vi "cleanPhaseSpaceData (SubVI).vi"(5 "raw trigger":dbl[][](array[numeric]), 7 "raw time":dbl[](array[numeric]), 8 "raw data":dbl[][](array[numeric])) -> (0 "data":waveform(dbl)[](array[waveform]), 1 "time stamp":dbl[](array[numeric]), 2 "stamped data":dbl[][](array[numeric]), 3 "raw data":dbl[][](array[numeric]), 4 "trigger PS":dbl[][](array[numeric]))   [LabVIEW 2017]
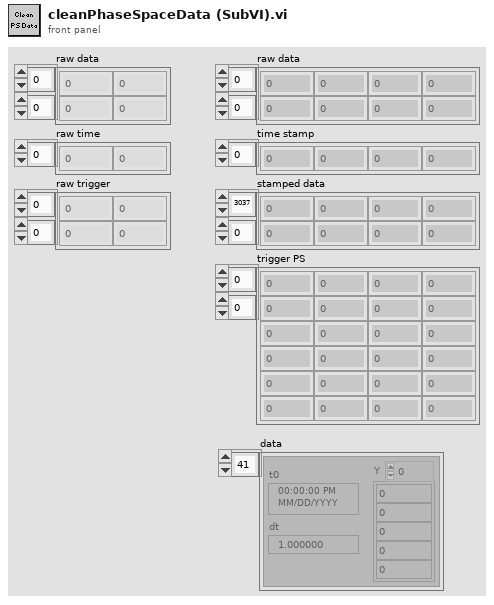
[diagram p1: front panel]
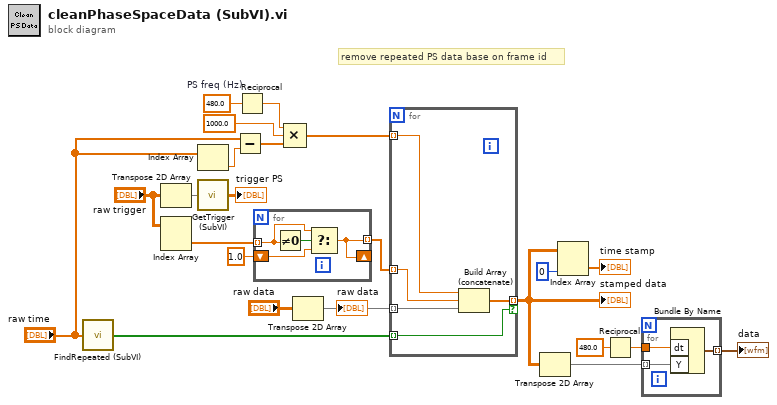
[diagram p0: block diagram]
diagram:
  w19 = 480.0  # PS freq (Hz)
  # "remove repeated PS data base on frame id"
  n1 = call "FindRepeated (SubVI).vi"("time stamp"="raw time") -> ("not repeated?"=w22:bool[])
  n2 = Transpose 2D Array(2D array="raw trigger") -> (transposed array=w14:dbl[][])
  n3 = Index Array(array="raw trigger") -> (element=w3:dbl[])  [unwired: 2 in]
  n4 = Index Array(array="raw time") -> (element=w17:dbl)  [unwired: 1 in]
  n5 = call "GetTrigger (SubVI).vi"("Array in"=w14) -> ("Array out"=→"trigger PS":dbl[][])  [unwired: 4 in]
  n6 = Subtract(x="raw time", y=w17) -> (x-y=w18:dbl[])
  n7 = Reciprocal(x=w19) -> (1/x=w20:dbl)
  n8 = for {
    tunnel: w3 -> [w26] mode=indexing
    shift-right: [w24] -> _
    shift-left: 1.0 -> [w25]
    tunnel: [w24] -> w1 mode=indexing
    n9 = Not Equal To 0?(x=w26) -> (x != 0?=w27:bool)
    n10 = Select(t=w26, s=w27, f=w25) -> (s? t:f=w24:dbl)
  }
  n11 = Compound Arithmetic op=MULTIPLY(w20, 1000.0 ("value"), w18) -> (w12:dbl[])
  n12 = Transpose 2D Array(2D array="raw data") -> (transposed array=w23:dbl[][])
  "raw data" <- w23
  n13 = for {
    tunnel: w23 -> [w29] mode=indexing
    tunnel: w22 -> [w28] mode=indexing
    tunnel: w12 -> [w32] mode=indexing
    tunnel: w1 -> [w31] mode=indexing
    tunnel: [w30] -> w5 mode=indexing if=w28
    n14 = Build Array (concatenate)(w32, w31, w29) -> (w30:dbl[])
  }
  "stamped data" <- w5
  n15 = Transpose 2D Array(2D array=w5) -> (transposed array=w6:dbl[][])
  n16 = Index Array(array=w5, index (col)=0 ("disabled index (col)")) -> (element=→"time stamp":dbl[])  [unwired: 1 in]
  n17 = Reciprocal(x=480.0 ("PS freq (Hz)")) -> (1/x=w7:dbl)
  n18 = for {
    tunnel: w6 -> [w35] mode=indexing
    tunnel: [w34] -> w4 mode=indexing
    tunnel: w7 -> [w33]
    n19 = Bundle By Name("dt"=w33, "Y"=w35) -> (w34:waveform(dbl))  [unwired: 1 in]
  }
  "data" <- w4
